vi "MPM_Get_READ_Power_for_Channel.vi"(8 "error in (no error)":errorcluster, 9 "channelNumber":i32, 10 "moduleNumber":i32, 11 ".NET Reference in":refnum<k24>) -> (0 "error out":errorcluster, 2 "power out":dbl, 3 "Reference out":refnum<k24>)   [LabVIEW 2017]
uses:
  C:/Users/Ssantec_Test/Documents/Instrument_DLL_Sample_Labview_20250826_Ver1.5.0_x64/DLL/InstrumentDLL.dll
  DLL/InstrumentDLL.dll
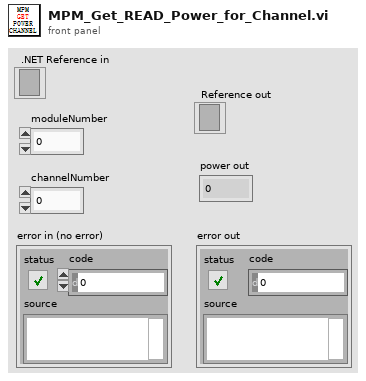
[diagram p1: front panel]
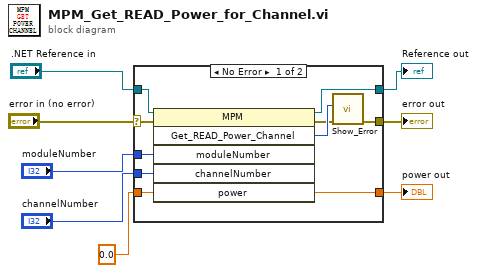
[diagram p0: block diagram]
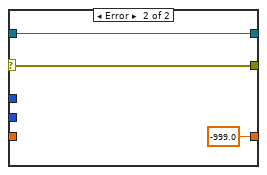
[diagram p2: hidden frame]
diagram:
  n1 = case shown="No Error" "error in (no error)" {
    selector: "error in (no error)" -> [w9 w20]
    tunnel: "channelNumber" -> [w18 _]
    tunnel: [w17 -999.0 ("power")] -> w7
    tunnel: "moduleNumber" -> [w16 _]
    tunnel: ".NET Reference in" -> [w15 w21]
    tunnel: [w14 w21] -> w4
    tunnel: 0.0 ("power") -> [w13 _]
    tunnel: [w10 w20] -> w2
    frame No Error {
      n2 = invoke on="调用节点" class="MPM" method="Get_READ_Power_Channel"(reference=w15, error in=w9, "moduleNumber"=w16, "channelNumber"=w18, "power"=w13) -> (reference out=w14:refnum<k24>, error out=w11:errorcluster, "Get_READ_Power_Channel"=w12:i32, "power"=w17:dbl)  [unwired: 1 in, 2 out]
      n3 = call "Show_Error.vi"("error in (no error)"=w11, "Error"=w12) -> ("error out"=w10:errorcluster)  [unwired: 9 in]
    }
    frame Error {
    }
  }
  "power out" <- w7
  "Reference out" <- w4
  "error out" <- w2
